vi "convertMilliMeterToEncoderUnits.vi"(8 "error in (no error)":errorcluster, 10 "Value In mm":dbl, 11 "Axis in":refnum<class "Axis.lvclass">) -> (0 "error out":errorcluster, 2 "Value In Encoder Units":dbl, 3 "Axis out":refnum<class "Axis.lvclass">)   [LabVIEW 2019, in "Axis.lvclass"]
uses:
  Axis.lvclass
  Axis.lvclass/Axis.ctl
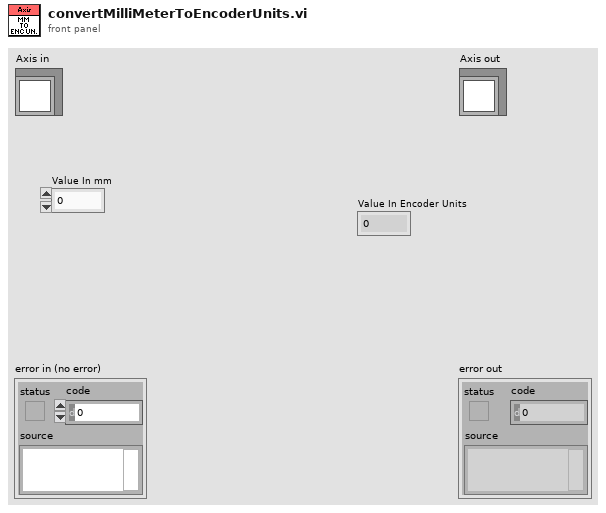
[diagram p1: front panel]
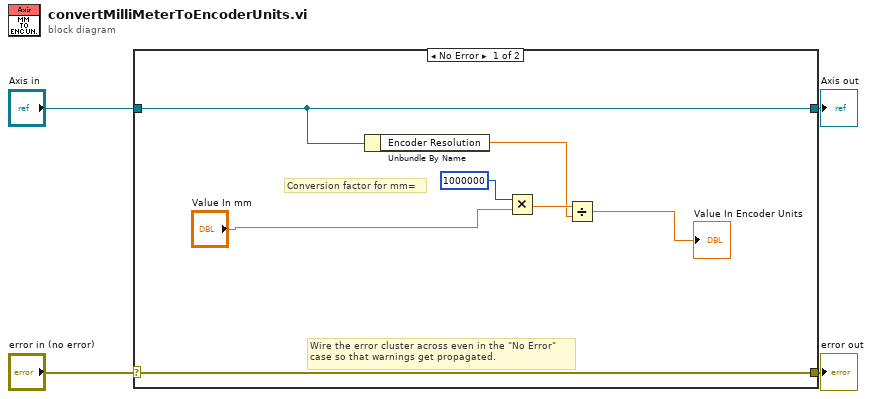
[diagram p0: block diagram]
diagram:
  n1 = case shown="No Error" "error in (no error)" {
    selector: "error in (no error)" -> [w11 w13]
    tunnel: [w11 w13] -> w3
    tunnel: [w8 w12] -> w1
    tunnel: "Axis in" -> [w8 w12]
    frame No Error {
      # "Conversion factor for mm="
      # "Wire the error cluster across even in the \"No Error\"\ncase so that warnings get propagated."
      n2 = Unbundle By Name(w8) -> ("Encoder Resolution"=w9:dbl)
      n3 = Multiply(x=1000000, y="Value In mm") -> (x*y=w10:dbl)
      n4 = Divide(x=w10, y=w9) -> (x/y=→"Value In Encoder Units":dbl)
    }
    frame Error {
    }
  }
  "error out" <- w3
  "Axis out" <- w1
